vi "Hi-Tech-Color-Senser_Read-Data.vi"() -> ()   [LabVIEW 2019]
uses:
  <vilib>/vision/NI_Vision_Development_Module.lvlib
panel:
  in  "Color Mode":u16(ring) items=["RGB", "HSL", "HSV", "HSI", "CIE L*a*b*", "CIE XYZ"]
  out "min(x,y)":T1
  out "max(x,y)":T1
  out "All Info":T1
  in  "Stop":bool
  out "Color":u32(colorbox)
  in  "Error In":errorcluster
  out "Error Out":errorcluster
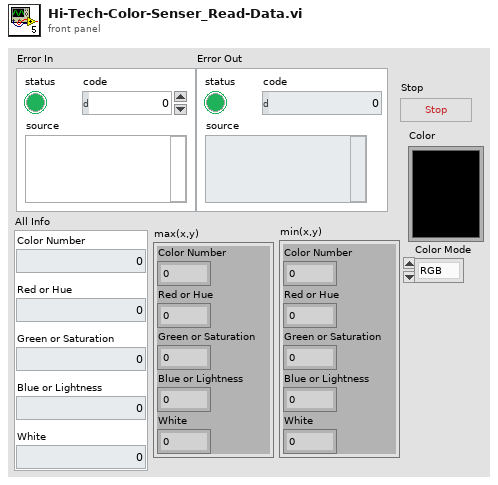
[diagram p1: front panel]
types:
  T1 = cluster{"Color Number":i32, "Red or Hue":i32, "Green or Saturation":i32, "Blue or Lightness":i32, "White":i32}
  T2 = typedef "I2C.lvlib/I2C Reference.ctl" = cluster{"myRIO Reference":T3, "I2C Channels Enum":T7, "I2C Configuration":T8}
  T3 = typedef "myRIO Generic Hardware Reference.ctl" = cluster{"myRIO Model":T4, "myRIO Hardware Reference":T5}
  T4 = typedef "Hardware Version Enum.ctl" = enum16{"Unknown", "myRIO-1900", "myRIO-1950", "roboRIO", "NI ELVIS RIO CM", "ELVIS III"}
  T5 = typedef "myRIO v1.0 Reference.ctl" = cluster{"Generic FPGA Reference":T6, "Allow multiple opens":bool}
  T6 = typedef "Generic FPGA Reference.ctl" = refnum<k20>
  T7 = typedef "I2C Channels Enum.ctl" = enum16{"Not Connected", "A/I2C", "B/I2C", "I2C/I2C"}
  T8 = typedef "I2C.lvlib/I2C Configuration.ctl" = cluster{"I2C Transfer Rate":T9}
  T9 = typedef "I2C.lvlib/I2C Transfer Rate.ctl" = enum16{"Standard mode (100 kbps)", "Fast mode (400 kbps)"}
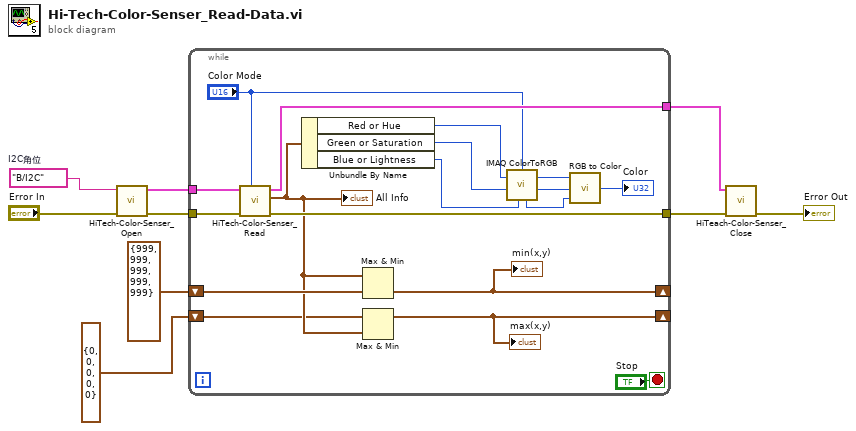
[diagram p0: block diagram]
diagram:
  w8 = tag "B/I2C"  # I2C角位
  n1 = call "HiTech-Color-Senser_Open.vi"("Error In"="Error In", "I2C角位"=w8) -> ("Error Out"=w9:errorcluster, "HiTechnicColorSensorV2 Ref Out"=w6:cluster{"I2C Ref Out":T2})  [unwired: 8 in]
  n2 = while {
    tunnel: w9 -> [w27]
    tunnel: w6 -> [w19]
    tunnel: [w18] -> w5
    tunnel: [w17] -> w4
    shift-right: [w15] -> _
    shift-left: T1 {"Color Number"=999, "Red or Hue"=999, "Green or Saturation"=999, "Blue or Lightness"=999, "White"=999} -> [w13]
    shift-right: [w14] -> _
    shift-left: T1 {"Color Number"=0, "Red or Hue"=0, "Green or Saturation"=0, "Blue or Lightness"=0, "White"=0} -> [w11]
    stop <- "Stop" stop-if-true
    n3 = call "HiTech-Color-Senser_Read.vi"("Color Mode"="Color Mode", "Error In"=w27, "HiTechnicColorSensorV2 Ref In"=w19) -> ("Error Out"=w17:errorcluster, "All Info"=w12:T1, "HiTechnicColorSensorV2 Ref Out"=w18:cluster{"I2C Ref Out":T2})  [unwired: 6 in]
    "All Info" <- w12
    n4 = Unbundle By Name(w12) -> ("Red or Hue"=w25:i32, "Green or Saturation"=w24:i32, "Blue or Lightness"=w26:i32)
    n5 = Max & Min(x=w12, y=w13) -> (min(x,y)=w15:T1)  [unwired: 1 out]
    "min(x,y)" <- w15
    n6 = Max & Min(x=w11, y=w12) -> (max(x,y)=w14:T1)  [unwired: 1 out]
    "max(x,y)" <- w14
    n7 = call "IMAQ ColorToRGB"("Green or Sat value"=w24, "Blue or Luma or Val or Inten value"=w26, "Red or Hue value"=w25, "Color Mode"="Color Mode") -> ("Blue value"=w21:u8, "Green value"=w22:u8, "Red value"=w23:u8)  [unwired: 1 in, 1 out]
    n8 = call <vilib>:"RGB to Color.vi"("B"=w21, "G"=w22, "R"=w23) -> ("Color"=→"Color":u32)
  }
  n9 = call "HiTeach-Color-Senser_Close.vi"("Error In"=w4, "HiTechnicColorSensorV2 Ref"=w5) -> ("Error Out"=→"Error Out":errorcluster)  [unwired: 9 in]
